vi "resistanceCalculator.vi"(0 "VISA Refnum in":refnum<visa-resource-name>, 11 "error in (no error)":errorcluster) -> (1 "ICON":cluster{dbl, dbl}[](array[cluster]), 3 "stepICON":dbl, 4 "steps/button Array":dbl[][](array[numeric]), 6 "cycle":dbl, 8 "No Keys":bool, 10 "KeyCodeName":string[](array[string]), 12 "EQF1255":cluster{dbl, dbl}[](array[cluster]), 14 "stepEQF1255":dbl, 15 "error out":errorcluster)   [LabVIEW 2018]
uses:
  <vilib>/express/express arith-compare/Formula/XNode/ExpressFormulaBlockNode.xnode
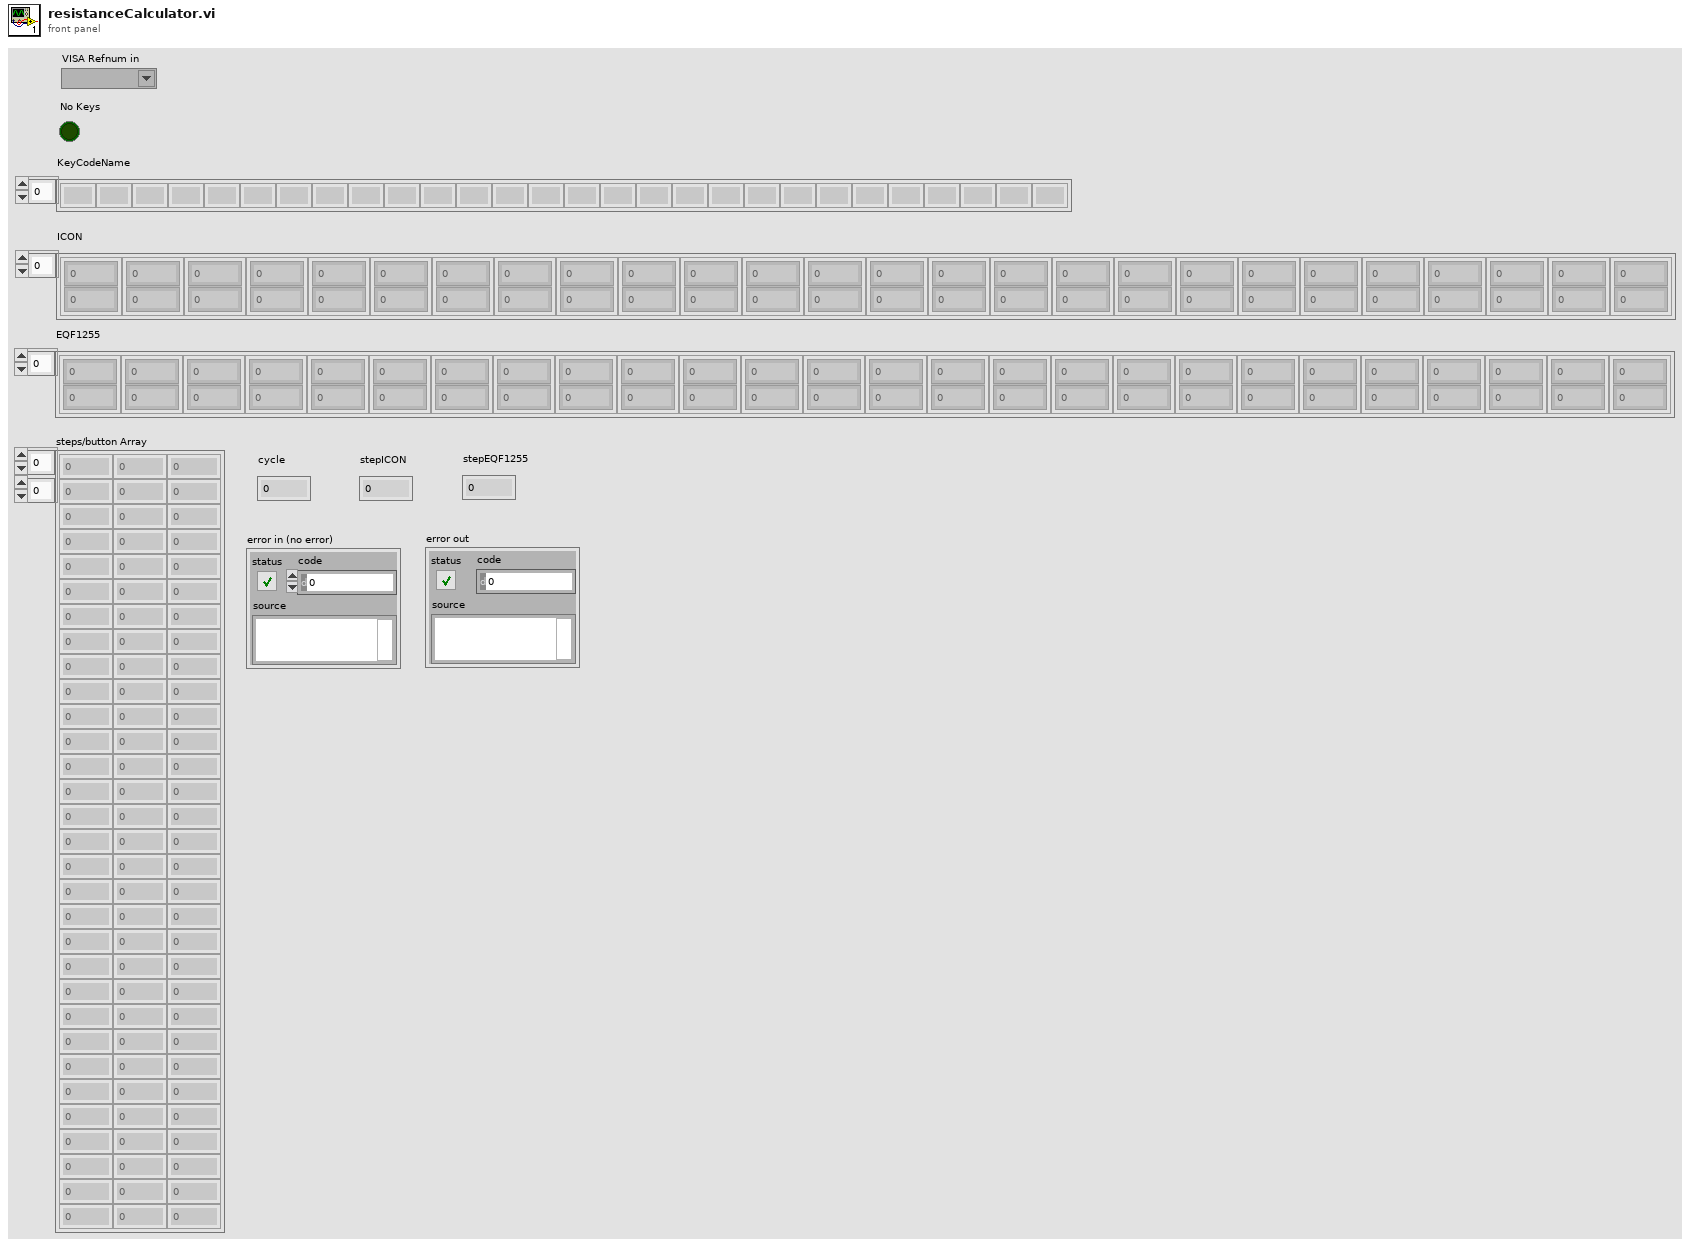
[diagram p1: front panel]
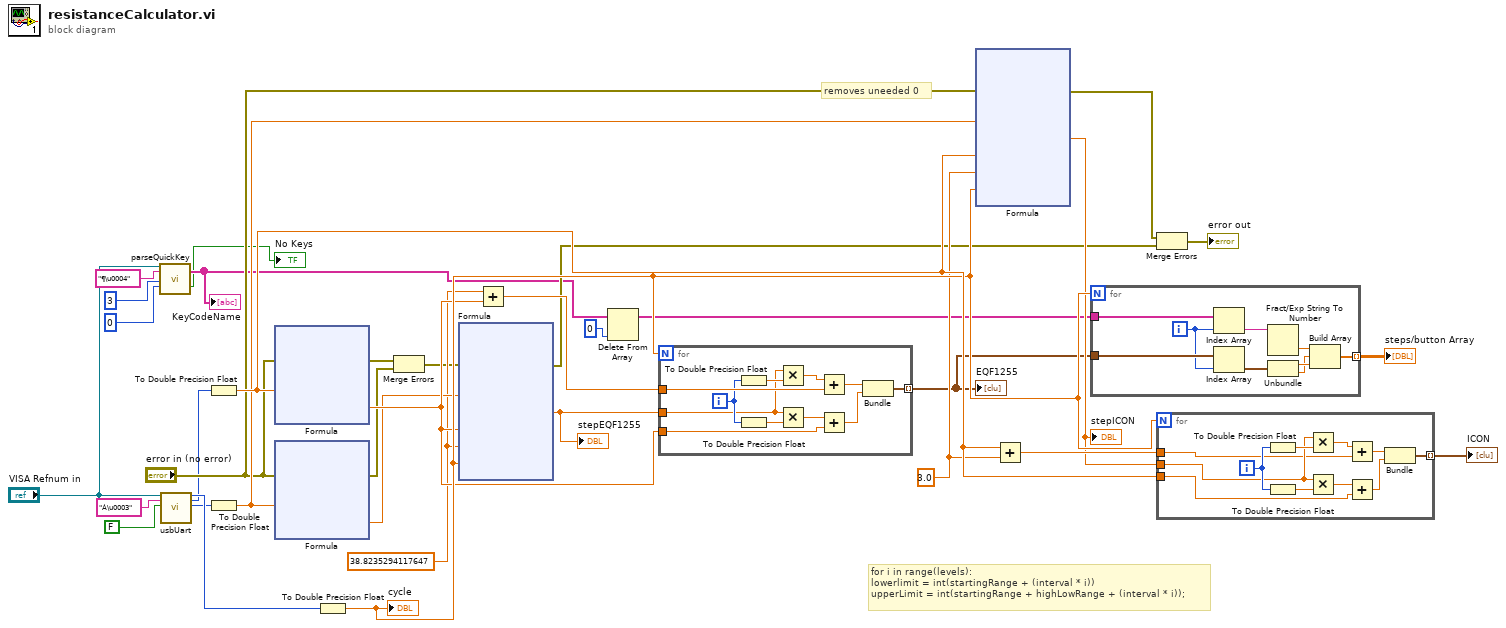
[diagram p0: block diagram]
diagram:
  w17 = 38.8235294117647
  w30 = 3.0 ("highlowRange")
  # "for i in range(levels):\nlowerlimit = int(startingRange + (interval * i))\nupperLimit = int(startingRange + highLowRange + (interval * i));"
  # "removes uneeded 0"
  n1 = call "parseQuickKey.vi"("VISA resource name"="VISA Refnum in", "write buffer"="¶\u0004", "y"=3, "x"=0 ("y")) -> ("KeyCodeName"=w8:string[], "No Keys"=→"No Keys":bool)  [unwired: 11 in, 3 out]
  "KeyCodeName" <- w8
  n2 = call "usbUart.vi"("VISA resource name"="VISA Refnum in", "write buffer"="Á\u0003", "sdFeature"=FALSE) -> ("number[0]"=w6:u32, "number[1]"=w5:u32, "number[2]"=w4:u32)  [unwired: 1 in, 13 out]
  n3 = To Double Precision Float(number=w5) -> (double precision float=w34:dbl)
  n4 = To Double Precision Float(number=w4) -> (double precision float=w32:dbl)
  n5 = xnode "Formula"("X1"=w34, "error in (no error)"="error in (no error)") -> ("Result"=w19:dbl, "error out"=w15:errorcluster)
  n6 = xnode "Formula"("X1"=w32, "error in (no error)"="error in (no error)") -> ("Result"=w18:dbl, "error out"=w14:errorcluster)
  n7 = To Double Precision Float(number=w6) -> (double precision float=w33:dbl)
  "cycle" <- w33
  n8 = Merge Errors(w15, w14) -> (w13:errorcluster)
  n9 = xnode "Formula"("max"=w18, "min"=w19, "range"=w17, "level"=w33, "error in (no error)"=w13) -> ("Result"=w16:dbl, "error out"=w11:errorcluster)
  "stepEQF1255" <- w16
  n10 = Add(x=w17, y=w19) -> (x+y=w20:dbl)
  n11 = Delete From Array(array=w8, index=0) -> (array with subset deleted=w26:string[])  [unwired: 1 in, 1 out]
  n12 = for {
    N: w33 -> [_]
    tunnel: w16 -> [w38]
    tunnel: w19 -> [w41]
    tunnel: w20 -> [w40]
    tunnel: [w37] -> w21 mode=indexing
    i -> [w39]
    n13 = To Double Precision Float(number=w39) -> (double precision float=w44:dbl)
    n14 = To Double Precision Float(number=w39) -> (double precision float=w43:dbl)
    n15 = Multiply(x=w38, y=w44) -> (x*y=w45:dbl)
    n16 = Multiply(x=w38, y=w43) -> (x*y=w42:dbl)
    n17 = Add(x=w45, y=w40) -> (x+y=w36:dbl)
    n18 = Add(x=w42, y=w41) -> (x+y=w35:dbl)
    n19 = Bundle(w36, w35) -> (w37:cluster{dbl, dbl})  [unwired: 1 in]
  }
  "EQF1255" <- w21
  n20 = xnode "Formula"("max"=w32, "min"=w34, "range"=w30, "level"=w33, "error in (no error)"="error in (no error)") -> ("Result"=w28:dbl, "error out"=w10:errorcluster)
  "stepICON" <- w28
  n21 = Add(x=w34, y=w30) -> (x+y=w31:dbl)
  n22 = for {
    N: w33 -> [_]
    tunnel: w21 -> [w54]
    tunnel: [w51] -> w27 mode=indexing
    tunnel: w26 -> [w48]
    i -> [w53]
    n23 = Index Array(array=w48, index=w53) -> (element=w47:string)
    n24 = Index Array(array=w54, index=w53) -> (element=w52:cluster{dbl, dbl})
    n25 = Fract/Exp String To Number(string=w47) -> (number=w46:dbl)  [unwired: 3 in, 1 out]
    n26 = Unbundle(w52) -> (w50:dbl, w49:dbl)
    n27 = Build Array(w46, w49, w50) -> (w51:dbl[])
  }
  "steps/button Array" <- w27
  n28 = Merge Errors(w10, w11) -> (→"error out":errorcluster)
  n29 = for {
    N: w33 -> [_]
    tunnel: w28 -> [w60]
    tunnel: [w59] -> w29 mode=indexing
    tunnel: w34 -> [w58]
    tunnel: w31 -> [w57]
    i -> [w61]
    n30 = To Double Precision Float(number=w61) -> (double precision float=w64:dbl)
    n31 = To Double Precision Float(number=w61) -> (double precision float=w63:dbl)
    n32 = Multiply(x=w60, y=w64) -> (x*y=w65:dbl)
    n33 = Multiply(x=w60, y=w63) -> (x*y=w62:dbl)
    n34 = Add(x=w65, y=w57) -> (x+y=w56:dbl)
    n35 = Add(x=w62, y=w58) -> (x+y=w55:dbl)
    n36 = Bundle(w56, w55) -> (w59:cluster{dbl, dbl})  [unwired: 1 in]
  }
  "ICON" <- w29
